vi "Update Engine Stream Filter IDs.vi"(8 "error in (no error)":errorcluster, 10 "IDs":u32[](array[numeric]), 11 "Refs":T1 {"Termination" items=["Off", "On"]}) -> (0 "error out":errorcluster)   [LabVIEW 2019, in "CAN Streaming Support Engine.lvlib"]
uses:
  CAN Streaming Support Engine.lvlib
  Types/Engine Stream API Refs.ctl
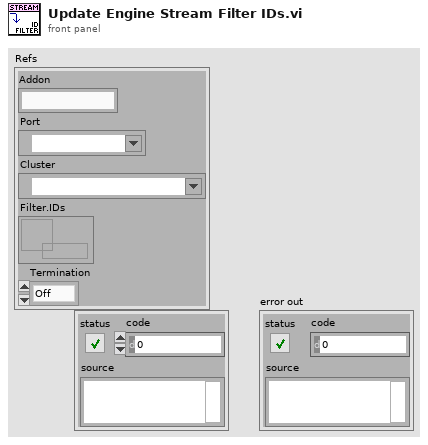
[diagram p1: front panel]
types:
  T1 = typedef "CAN Streaming Support Engine.lvlib/Engine Stream API Refs.ctl" = cluster{"Addon":string, "Port":refnum<k21>, "Cluster":refnum<k21>, "Filter.IDs":refnum<data-value>, "Termination":u32}
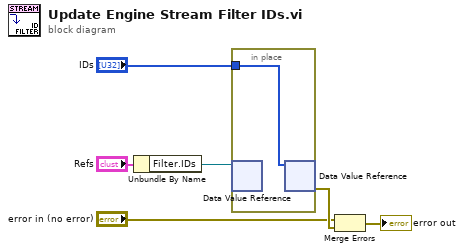
[diagram p0: block diagram]
diagram:
  n1 = Unbundle By Name("Refs") -> ("Filter.IDs"=w2:refnum<data-value>)
  n2 = in-place {
    in-place-border: "IDs" -> [w7]
    n3 = in-place-dvr #1(w2) -> ()  [unwired: 2 out]
    n4 = in-place-dvr #1(w7) -> (w5:errorcluster)  [unwired: 1 out]
  }
  n5 = Merge Errors("error in (no error)", w5) -> (→"error out":errorcluster)
